vi "Get Convex Polygon.vi"(9 "Convex Hull Points":i32[](array[numeric]), 10 "y":dbl[](array[numeric]), 11 "X":dbl[](array[numeric])) -> (2 "Y":dbl[](array[numeric]), 3 "X":dbl[](array[numeric]))   [LabVIEW 2014]
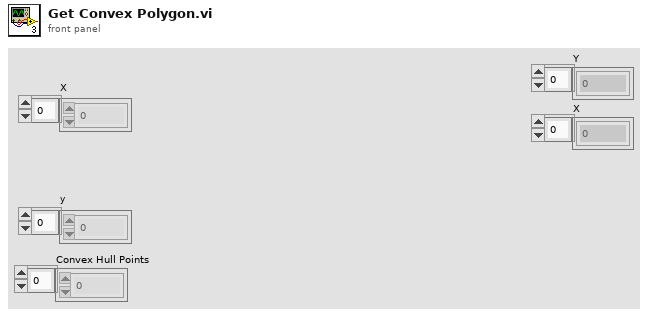
[diagram p1: front panel]
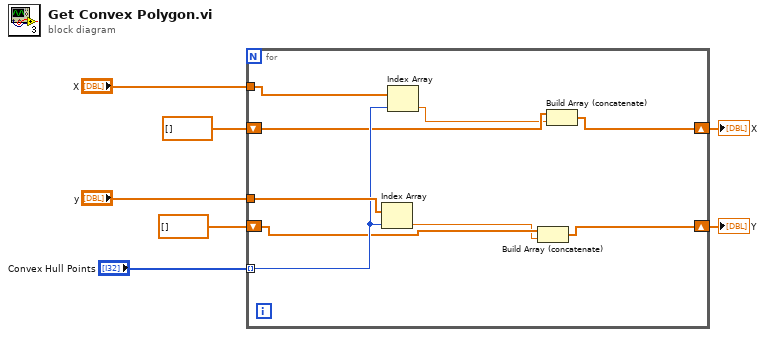
[diagram p0: block diagram]
diagram:
  n1 = for {
    tunnel: "Convex Hull Points" -> [w14] mode=indexing
    tunnel: "y" -> [w15]
    tunnel: "X" -> [w16]
    shift-right: [w9] -> w1
    shift-left: dbl[] [] -> [w11]
    shift-right: [w8] -> w2
    shift-left: dbl[] [] -> [w13]
    n2 = Index Array(array=w15, index=w14) -> (element=w12:dbl)
    n3 = Index Array(array=w16, index=w14) -> (element=w10:dbl)
    n4 = Build Array (concatenate)(w13, w12) -> (w8:dbl[])
    n5 = Build Array (concatenate)(w11, w10) -> (w9:dbl[])
  }
  "Y" <- w2
  "X" <- w1
